vi "Read ContexMenue.vi"(8 "error in (no error)":errorcluster, 11 "ContexMenue in":refnum<class "ContexMenue.lvclass">) -> (0 "error out":errorcluster, 2 "ContexMenue":refnum<k24>, 3 "ContexMenue out":refnum<class "ContexMenue.lvclass">)   [LabVIEW 2016, in "ContexMenue.lvclass"]
uses:
  ContexMenue.lvclass
  System.Windows.Forms
  ContexMenue.lvclass/ContexMenue.ctl
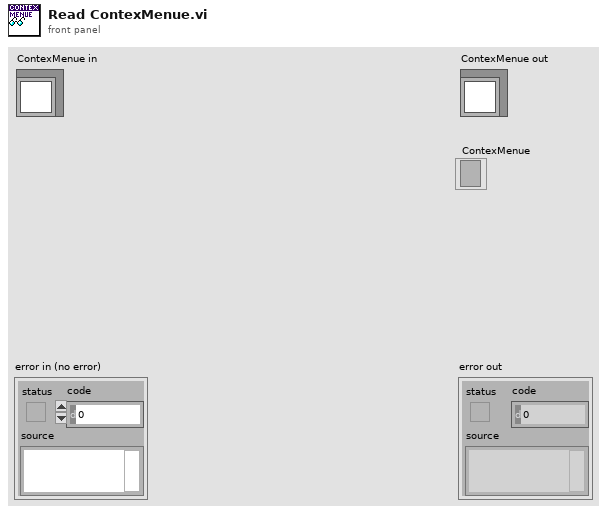
[diagram p1: front panel]
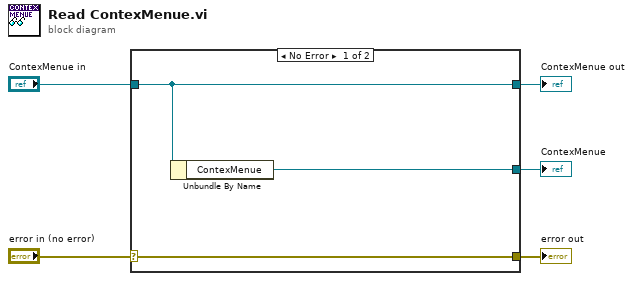
[diagram p0: block diagram]
diagram:
  n1 = case shown="No Error" "error in (no error)" {
    selector: "error in (no error)" -> [w8 w9]
    tunnel: [w8 w9] -> w4
    tunnel: [w7 w10] -> w2
    tunnel: "ContexMenue in" -> [w7 w10]
    tunnel: [w6 _] -> w1
    frame No Error {
      n2 = Unbundle By Name(w7) -> ("ContexMenue"=w6:refnum<k24>)
    }
    frame Error {
    }
  }
  "error out" <- w4
  "ContexMenue out" <- w2
  "ContexMenue" <- w1
